vi "FPGA_bubble_SCTL.vi"() -> ()   [LabVIEW 2020]
uses:
  <vilib>/Platform/TimedLoop/XDataNode/timing_clust.ctl
  <vilib>/Platform/TimedLoop/XDataNode/nitl_modes.ctl
  <vilib>/Platform/TimedLoop/XDataNode/wakeup.ctl
  <vilib>/platform/TimedLoop/XDataNode/XDataNode.xnode
  <vilib>/rvi/DataTransferAndStorage/Container/XNode/niFpgaContainer.xnode
  <vilib>/rvi/interface/RandomDataEmulation/nirviRandomDataFpgaReadWriteTemplate.vi
  <vilib>/rvi/FIFO/Fifo_Resource/nirvififoEmulationWrite.vi
  <vilib>/Platform/TimedLoop/XDataNode/XDNodeRunTimeDep.lvlib
panel:
  out "index Array":i32[](array[numeric])
  out "Output Valid":bool
  out "Sorted array":sgl[](array[numeric])
  out "Sorted index":u8[](array[numeric])
  in  "Input Array":sgl[](array[numeric])=[0.0, 0.0, 0.0, 0.0, 0.0, 0.0, 0.0, 0.0]
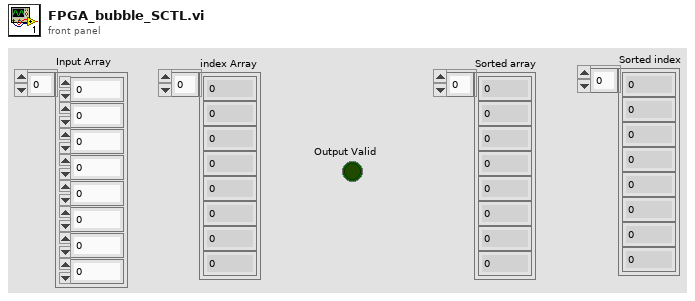
[diagram p1: front panel]
types:
  T1 = typedef "XDNodeRunTimeDep.lvlib/timing_clust.ctl" = cluster{"Expected End [f-1]":u64, "Actual End [f-1]":u64, "Finished Late? [f-1]":bool, "Expected End [i-1]":u64, "Actual End [i-1]":u64, "Finished Late? [i-1]":bool, "Expected Start [i]":u64, "Actual Start [i]":u64, "Expected Start [f]":u64, "Actual Start [f]":u64, "Source Name":string, "Structure Name":string, "Period":i64, "Deadline":i64, "Offset":i64, "Start":i64, "Priority":i32, "Timeout":i32, "Mode":T2, "Wakeup Reason":T3, "Error":errorcluster, "Source Type":string, "Secondary Source Type":string, "Global End Time":u64, "Global Start Time":u64, "Frame Duration":u64, "Iteration Duration":u64, "Assigned CPU":i32, "I/O Scan Engine Mode":u32}
  T2 = typedef "XDNodeRunTimeDep.lvlib/nitl_modes.ctl" = enum32{"No Change", "Process missed periods, maintain original phase", "Discard missed periods, maintain original phase", "Process missed periods, ignore original phase", "Discard missed periods, ignore original phase"}
  T3 = typedef "XDNodeRunTimeDep.lvlib/wakeup.ctl" = enum32{"Normal", "Aborted", "Asynchronous wakeup", "Timing source error", "Timed loop error", "Timeout"}
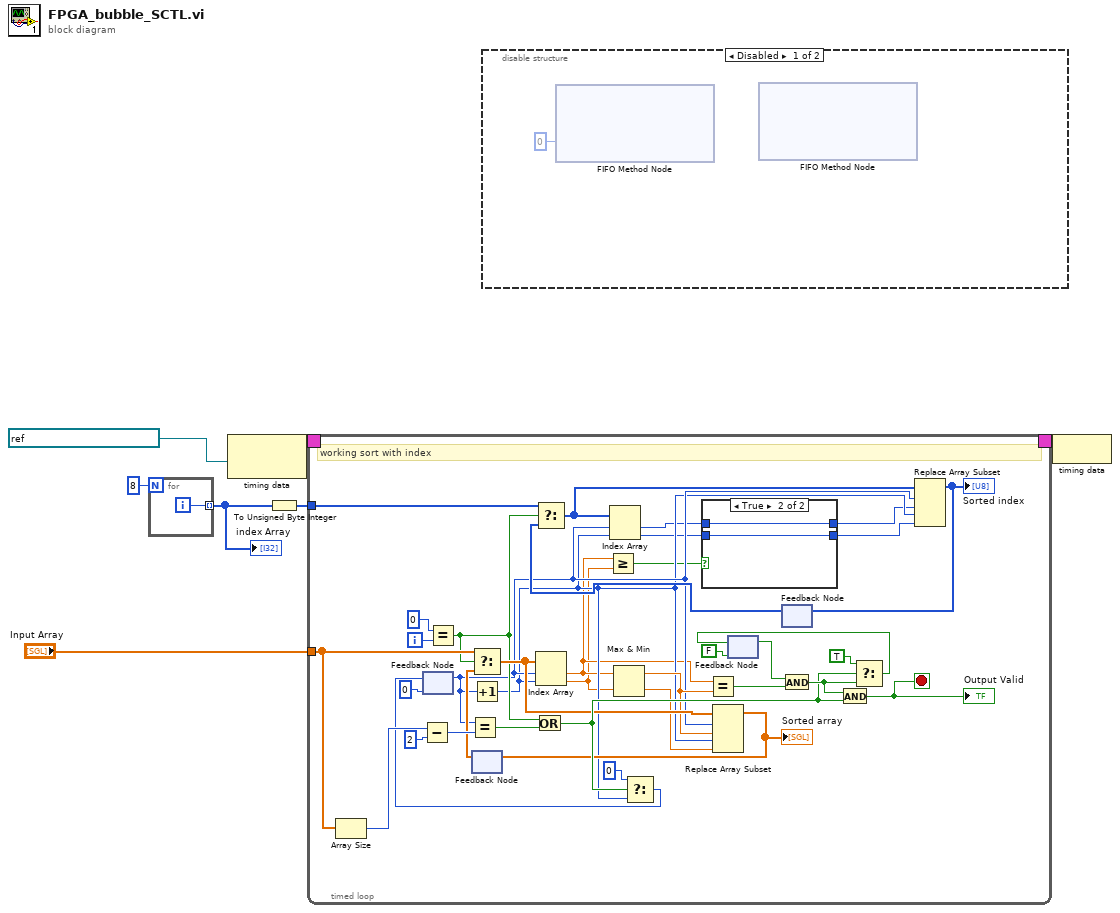
[diagram p0: block diagram]
diagram:
  n1 = for {
    N: 8 -> [_]
    tunnel: [w8] -> w6 mode=indexing
    i -> [w8]
  }
  "index Array" <- w6
  n2 = node-c288(refnum<k21> "40 MHz Onboard Clock" ("Source Name")) -> (w3:T1)
  n3 = To Unsigned Byte Integer(number=w6) -> (unsigned 8bit integer=w5:u8[])
  n4 = timed-loop {
    tunnel: "Input Array" -> [w42]
    tunnel: w5 -> [w20]
    timing: w3 -> [_]
    timing-out: [_] -> w2
    i -> [w24]
    stop <- w25 stop-if-true
    # "working sort with index"
    n5 = Array Size(array=w42) -> (size(s)=w45:i32)
    n6 = Subtract(x=w45, y=2) -> (x-y=w43:i32)
    n7 = feedback #1(0 ("y")) -> (w18:i32)
    n8 = Equal?(x=0, y=w24) -> (x = y?=w19:bool)
    n9 = Equal?(x=w18, y=w43) -> (x = y?=w30:bool)
    n10 = Increment(x=w18) -> (x+1=w17:i32)
    n11 = feedback #2() -> (w35:sgl[])  [unwired: 1 in]
    n12 = Select(t=w42, s=w19, f=w35) -> (s? t:f=w29:sgl[])
    n13 = Or(x=w19, y=w30) -> (x .or. y?=w33:bool)
    n14 = Index Array(array=w29, index #1=w18, index #2=w17) -> (element #1=w11:sgl, element #2=w10:sgl)
    n15 = Greater Or Equal?(x=w11, y=w10) -> (x >= y?=w9:bool)
    n16 = Max & Min(x=w11, y=w10) -> (max(x,y)=w27:sgl, min(x,y)=w26:sgl)
    n17 = Select(t=0 ("y"), s=w33, f=w17) -> (s? t:f=w31:i32)
    n18 = feedback-in #1(w31) -> ()
    n19 = Equal?(x=w11, y=w27) -> (x = y?=w41:bool)
    n20 = Replace Array Subset(array=w29, new element #1=w27, index #1=w18, new element #2=w26, index #2=w17) -> (w28:sgl[])
    "Sorted array" <- w28
    n21 = feedback-in #2(w28) -> ()
    n22 = feedback #3(FALSE ("t")) -> (w38:bool)
    n23 = feedback #4() -> (w22:u8[])  [unwired: 1 in]
    n24 = Select(t=w20, s=w19, f=w22) -> (s? t:f=w21:u8[])
    n25 = Index Array(array=w21, index #1=w18, index #2=w17) -> (element #1=w15:u8, element #2=w12:u8)
    n26 = case shown="True" w9 {
      tunnel: w15 -> [w47 w49]
      tunnel: [w46 w49] -> w14
      tunnel: [w47 w48] -> w13
      tunnel: w12 -> [w46 w48]
      frame False {
      }
      frame True {
      }
    }
    n27 = And(x=w38, y=w41) -> (x .and. y?=w36:bool)
    n28 = And(x=w36, y=w33) -> (x .and. y?=w25:bool)
    "Output Valid" <- w25
    n29 = Select(t=TRUE, s=w33, f=w36) -> (s? t:f=w39:bool)
    n30 = feedback-in #3(w39) -> ()
    n31 = Replace Array Subset(array=w21, new element #1=w14, index #1=w18, new element #2=w13, index #2=w17) -> (w16:u8[])
    "Sorted index" <- w16
    n32 = feedback-in #4(w16) -> ()
  }
  n33 = disable-structure shown="Disabled" {
    frame Disabled {
      n34 = xnode ("FIFO Method Node")("Timeout"=0) -> ()  [unwired: 1 in, 3 out]
      n35 = xnode ("FIFO Method Node")() -> ()  [unwired: 3 in, 2 out]
    }
    frame Enabled {
    }
  }
  n36 = node-c288(w2) -> ()
